vi "Auto Stack.vi"(11 "Button":bool) -> ()   [LabVIEW 2014]
uses:
  <vilib>/Rock Robotics/WPI/Solenoid/Deprecated/WPI_SolenoidSetBool.vi
panel:
  out "Top":dbl
  out "Middle":dbl
  out "Bottom":dbl
  in  "Boolean":bool
  in  "Last Fed Value":dbl
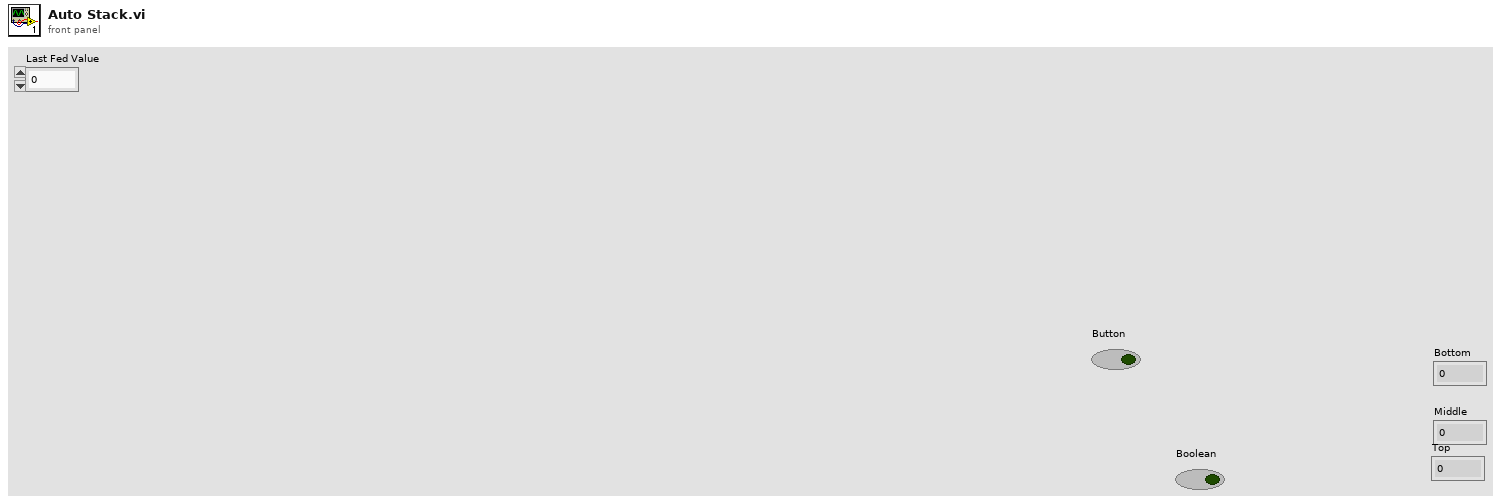
[diagram p1: front panel]
types:
  T1 = typedef "WPI_MotorControlDeviceRef.ctl" = cluster{"DeviceStatus":errorcluster, "Type":T2, "PWM":cluster{"Controller":T3, "PWM Channel":T4, "DeadBand":T5}, "CAN":cluster{"Device Number":u8, "Control Mode":T6, "Semaphore":T7, "Max Vout":dbl, "TalonSRX Control Mode":T8}, "Invert":bool, "TransformRef":T9, "InvTransformRef":T9}
  T2 = typedef "WPI_MotorControlType.ctl" = enum16{"PWM", "CAN", "CANTalonSRX"}
  T3 = typedef "FPGA_TypedefDigitalModule.ctl" = enum16{"Controller 1"}
  T4 = typedef "FPGA_DIOPWMChannel.ctl" = enum8{"PWM 0", "PWM 1", "PWM 2", "PWM 3", "PWM 4", "PWM 5", "PWM 6", "PWM 7", "PWM 8", "PWM 9", "PWM MXP 0", "PWM MXP 1", "PWM MXP 2", "PWM MXP 3", "PWM MXP 4", "PWM MXP 5", "PWM MXP 6", "PWM MXP 7", "PWM MXP 8", "PWM MXP 9", "Invalid"}
  T5 = typedef "WPI_PWMDeadband.ctl" = cluster{"Name":string, "maxPositivePwm":i32, "minPositivePwm":i32, "centerPwm":i32, "maxNegativePwm":i32, "minNegativePwm":i32, "angularRange":u16}
  T6 = typedef "WPI_CANJaguar_ControlMode.ctl" = enum8{"Percent VBus", "Current", "Speed", "Position", "Voltage"}
  T7 = typedef "Semaphore RefNum" = refnum<k1>
  T8 = typedef "WPI_CANTalonSRX_APIControlMode.ctl" = enum8{"Percent VBus", "Speed", "Position", "Slave", "Unchanged / Invalid"}
  T9 = typedef "WPI_PWMTransform_ConPane.ctl" = refnum<vi>
  T10 = typedef "WPI_AnalogChannelDevRef.ctl" = cluster{"DevStatus":errorcluster, "Controller":T11, "Analog Channel":T12}
  T11 = typedef "FPGA_TypedefAnalogModule.ctl" = enum16{"Controller 1"}
  T12 = typedef "FPGA_AIChannel.ctl" = enum8{"AI 0", "AI 1", "AI 2", "AI 3", "AI MXP 0", "AI MXP 1", "AI MXP 2", "AI MXP 3", "Invalid"}
  T13 = typedef "WPI_PotentiometerDevRef.ctl" = cluster{"DevStatus":errorcluster, "Controller":T11, "Analog Channel":T12, "Invert Output":bool}
  T14 = typedef "WPI_SolenoidDevRef.ctl" = cluster{"DevStatus":errorcluster, "Pneumatics Control Module":u8, "Forward Solenoid Channel":T15, "Reverse Solenoid Channel":T15}
  T15 = typedef "WPI_SolenoidChannel.ctl" = enum8{"Solenoid 0", "Solenoid 1", "Solenoid 2", "Solenoid 3", "Solenoid 4", "Solenoid 5", "Solenoid 6", "Solenoid 7", "Invalid"}
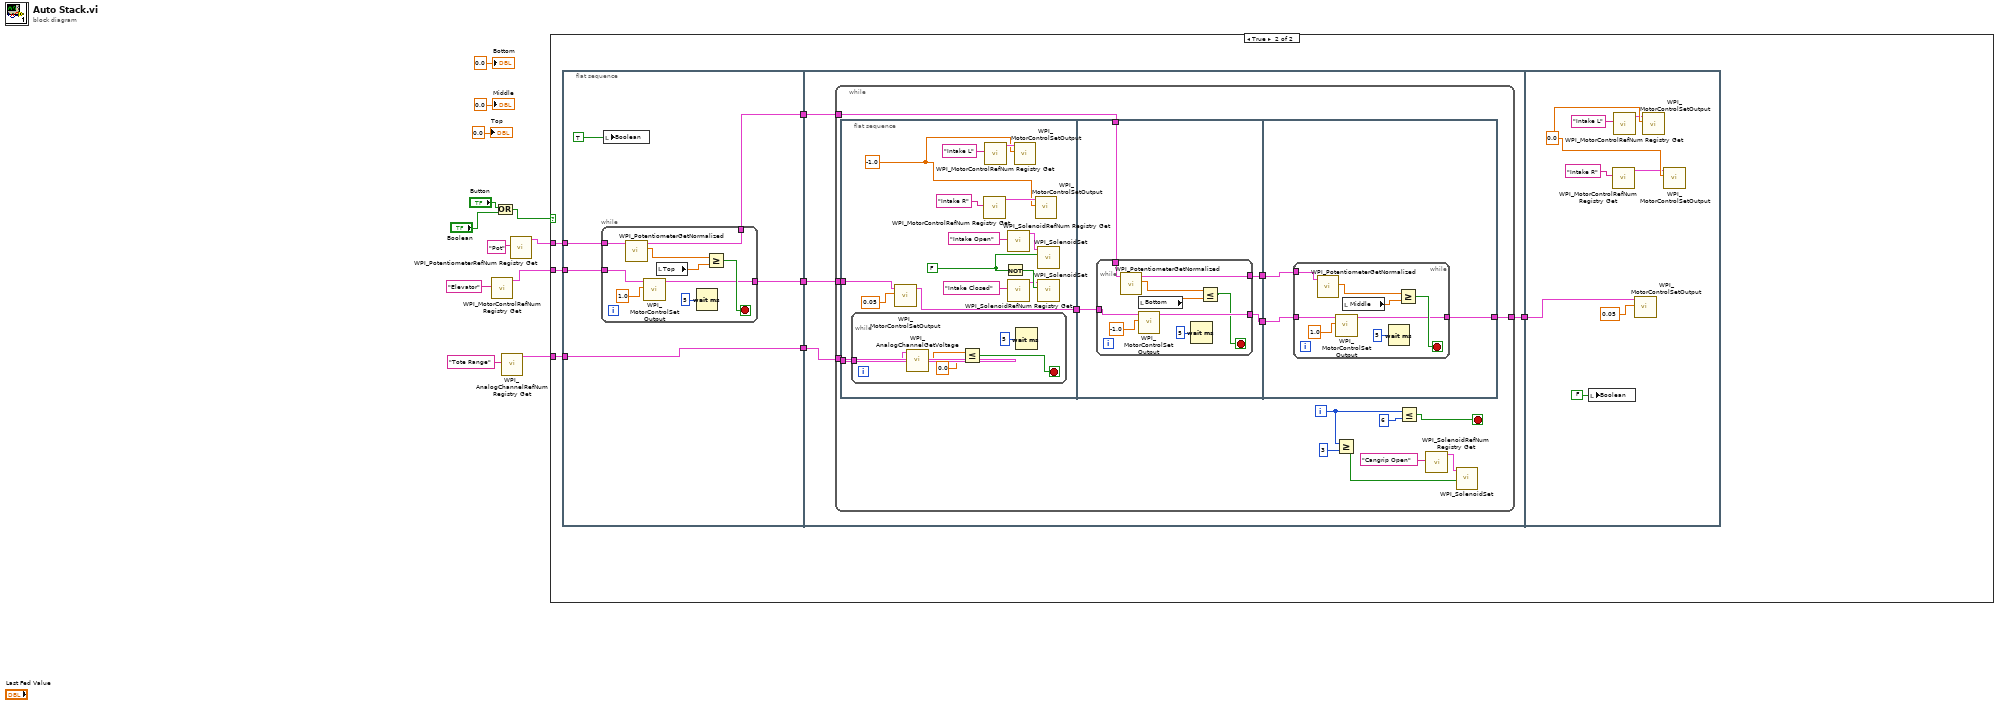
[diagram p0: block diagram]
diagram:
  n1 = call <vilib>:"WPI_MotorControlRefNum Registry Get.vi"("refnum name"="Elevator") -> ("MotorControlDevRef"=w8:T1)  [unwired: 9 in, 1 out]
  n2 = Or(x="Button", y="Boolean") -> (x .or. y?=w10:bool)
  n3 = call <vilib>:"WPI_AnalogChannelRefNum Registry Get.vi"("refnum name"="Tote Range") -> ("AIDeviceRef"=w1:T10)  [unwired: 9 in, 1 out]
  n4 = call <vilib>:"WPI_PotentiometerRefNum Registry Get.vi"("refnum name"="Pot") -> ("PotDevRef"=w6:T13)  [unwired: 9 in, 1 out]
  n5 = case shown="True" w10 {
    tunnel: w8 -> [_ w19]
    tunnel: w6 -> [_ w18]
    tunnel: w1 -> [_ w16]
    frame False {
    }
    frame True {
      n6 = flat-sequence {
        tunnel: w19 -> [w25]
        tunnel: w18 -> [w24]
        tunnel: [w22] -> w17
        tunnel: w16 -> [w22]
        tunnel: [w21] -> w15
        tunnel: [w20] -> w14
        tunnel: w17 -> [w38]
        tunnel: w15 -> [w37]
        tunnel: w14 -> [w36]
        tunnel: [w35] -> w13
        tunnel: w13 -> [w98]
        frame #0 {
          n7 = while {
            tunnel: w25 -> [w33]
            tunnel: w24 -> [w32]
            tunnel: [w27] -> w21
            tunnel: [w26] -> w20
            stop <- w29 stop-if-true
            n8 = call <vilib>:"WPI_PotentiometerGetNormalized.vi"("PotDevRef"=w32) -> ("Normalized Value"=w31:dbl, "PotDevRef"=w26:T13)  [unwired: 8 in, 1 out]
            n9 = call <vilib>:"WPI_MotorControlSetOutput.vi"("Output"=1.0, "MotorControlDevRef"=w33) -> ("MotorControlDevRef"=w27:T1)  [unwired: 7 in, 2 out]
            n10 = local read "Top"() -> (w30:dbl)
            n11 = Wait (ms)(milliseconds to wait=u32 5) -> ()  [unwired: 1 out]
            n12 = Greater Or Equal?(x=w31, y=w30) -> (x >= y?=w29:bool)
          }
          n13 = local write "Boolean"(TRUE) -> ()
        }
        frame #1 {
          n14 = while {
            tunnel: w38 -> [w52]
            tunnel: w37 -> [w49]
            tunnel: w36 -> [w48]
            tunnel: [w44] -> w35
            i -> [w41]
            stop <- w51 stop-if-true
            n15 = flat-sequence {
              tunnel: w52 -> [w67]
              tunnel: w49 -> [w65]
              tunnel: [w53] -> w46
              tunnel: w48 -> [w76]
              tunnel: [w75] -> w47
              tunnel: w46 -> [w74]
              tunnel: [w73] -> w45
              tunnel: w47 -> [w88]
              tunnel: w45 -> [w87]
              tunnel: [w86] -> w44
              frame #0 {
                w54 = FALSE
                w60 = -1.0 ("Output")
                n16 = while {
                  tunnel: w67 -> [w68]
                  stop <- w70 stop-if-true
                  n17 = call <vilib>:"WPI_AnalogChannelGetVoltage.vi"("AIDeviceRef"=w68) -> ("Voltage"=w72:dbl)  [unwired: 8 in, 2 out]
                  n18 = Less Or Equal?(x=w72, y=0.0) -> (x <= y?=w70:bool)
                  n19 = Wait (ms)(milliseconds to wait=u32 5) -> ()  [unwired: 1 out]
                }
                n20 = call <vilib>:"WPI_MotorControlSetOutput.vi"("Output"=0.05, "MotorControlDevRef"=w65) -> ("MotorControlDevRef"=w53:T1)  [unwired: 7 in, 2 out]
                n21 = call <vilib>:"WPI_MotorControlRefNum Registry Get.vi"("refnum name"="Intake R") -> ("MotorControlDevRef"=w62:T1)  [unwired: 9 in, 1 out]
                n22 = call <vilib>:"WPI_MotorControlRefNum Registry Get.vi"("refnum name"="Intake L") -> ("MotorControlDevRef"=w61:T1)  [unwired: 9 in, 1 out]
                n23 = Not(x=w54) -> (.not. x?=w59:bool)
                n24 = call <vilib>:"WPI_SolenoidRefNum Registry Get.vi"("refnum name"="Intake Open") -> ("SolenoidDevRef"=w56:T14)  [unwired: 9 in, 1 out]
                n25 = call <vilib>:"WPI_SolenoidRefNum Registry Get.vi"("refnum name"="Intake Closed") -> ("SolenoidDevRef"=w57:T14)  [unwired: 9 in, 1 out]
                n26 = call <vilib>:"WPI_MotorControlSetOutput.vi"("Output"=w60, "MotorControlDevRef"=w61) -> ()  [unwired: 7 in, 3 out]
                n27 = call <vilib>:"WPI_MotorControlSetOutput.vi"("Output"=w60, "MotorControlDevRef"=w62) -> ()  [unwired: 7 in, 3 out]
                n28 = call-poly <vilib>:"WPI_SolenoidSet.vi"("Value"=w54, "SolenoidDevRef"=w56) -> ()  [unwired: 8 in, 2 out]
                n29 = call-poly <vilib>:"WPI_SolenoidSet.vi"("Value"=w59, "SolenoidDevRef"=w57) -> ()  [unwired: 8 in, 2 out]
              }
              frame #1 {
                n30 = while {
                  tunnel: [w83] -> w73
                  tunnel: w76 -> [w82]
                  tunnel: [w81] -> w75
                  tunnel: w74 -> [w80]
                  stop <- w79 stop-if-true
                  n31 = call <vilib>:"WPI_PotentiometerGetNormalized.vi"("PotDevRef"=w82) -> ("Normalized Value"=w78:dbl, "PotDevRef"=w81:T13)  [unwired: 8 in, 1 out]
                  n32 = local read "Bottom"() -> (w77:dbl)
                  n33 = call <vilib>:"WPI_MotorControlSetOutput.vi"("Output"=-1.0, "MotorControlDevRef"=w80) -> ("MotorControlDevRef"=w83:T1)  [unwired: 7 in, 2 out]
                  n34 = Wait (ms)(milliseconds to wait=u32 5) -> ()  [unwired: 1 out]
                  n35 = Less Or Equal?(x=w78, y=w77) -> (x <= y?=w79:bool)
                }
              }
              frame #2 {
                n36 = while {
                  tunnel: [w92] -> w86
                  tunnel: w88 -> [w91]
                  tunnel: w87 -> [w90]
                  stop <- w94 stop-if-true
                  n37 = call <vilib>:"WPI_PotentiometerGetNormalized.vi"("PotDevRef"=w91) -> ("Normalized Value"=w95:dbl)  [unwired: 8 in, 2 out]
                  n38 = call <vilib>:"WPI_MotorControlSetOutput.vi"("Output"=1.0, "MotorControlDevRef"=w90) -> ("MotorControlDevRef"=w92:T1)  [unwired: 7 in, 2 out]
                  n39 = local read "Middle"() -> (w89:dbl)
                  n40 = Wait (ms)(milliseconds to wait=u32 5) -> ()  [unwired: 1 out]
                  n41 = Greater Or Equal?(x=w95, y=w89) -> (x >= y?=w94:bool)
                }
              }
            }
            n42 = Greater Or Equal?(x=w41, y=3) -> (x >= y?=w40:bool)
            n43 = Less Or Equal?(x=w41, y=6) -> (x <= y?=w51:bool)
            n44 = call <vilib>:"WPI_SolenoidRefNum Registry Get.vi"("refnum name"="Cangrip Open") -> ("SolenoidDevRef"=w43:T14)  [unwired: 9 in, 1 out]
            n45 = call-poly <vilib>:"WPI_SolenoidSet.vi"("Value"=w40, "SolenoidDevRef"=w43) -> ()  [unwired: 8 in, 2 out]
          }
        }
        frame #2 {
          w104 = 0.0 ("Output")
          n46 = local write "Boolean"(FALSE ("Boolean")) -> ()
          n47 = call <vilib>:"WPI_MotorControlRefNum Registry Get.vi"("refnum name"="Intake R") -> ("MotorControlDevRef"=w102:T1)  [unwired: 9 in, 1 out]
          n48 = call <vilib>:"WPI_MotorControlRefNum Registry Get.vi"("refnum name"="Intake L") -> ("MotorControlDevRef"=w103:T1)  [unwired: 9 in, 1 out]
          n49 = call <vilib>:"WPI_MotorControlSetOutput.vi"("Output"=0.05, "MotorControlDevRef"=w98) -> ()  [unwired: 7 in, 3 out]
          n50 = call <vilib>:"WPI_MotorControlSetOutput.vi"("Output"=w104, "MotorControlDevRef"=w103) -> ()  [unwired: 7 in, 3 out]
          n51 = call <vilib>:"WPI_MotorControlSetOutput.vi"("Output"=w104, "MotorControlDevRef"=w102) -> ()  [unwired: 7 in, 3 out]
        }
      }
    }
  }
  "Bottom" <- 0.0 ("Bottom")
  "Middle" <- 0.0 ("Middle")
  "Top" <- 0.0 ("Middle")
